vi "Velocidad con Perfiles.vi"() -> ()   [LabVIEW 2014]
uses:
  <vilib>/LabVIEW Interface for Arduino/Type Defs/Pin Mode.ctl
  <vilib>/LabVIEW Interface for Arduino/LabVIEW Interface for Arduino.lvlib
panel:
  out "Boolean 4":bool
  out "Boolean 3":bool
  out "Boolean 2":bool
  out "Boolean":bool
  in  "Enum":enum16{"Detenido", "Baja", "Media", "Alta"}(ring)
  in  "VISA resource name":refnum<visa-resource-name>
  # "Recurso"
  # "Velocidad"
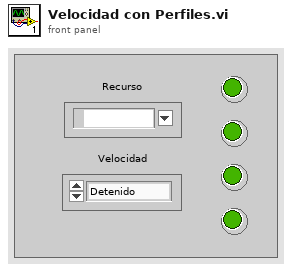
[diagram p1: front panel]
types:
  T1 = typedef "LabVIEW Interface for Arduino.lvlib/Pin Mode.ctl" = enum8{"Input", "Output"}
  T2 = typedef "LabVIEW Interface for Arduino.lvlib/Arduino Resource.ctl" = cluster{"VISA resource":refnum<visa-resource-name>, "Board Type":T3, "Connection Type":enum8{"USB / Serial"}, "Bytes Per Packet (15)":u8}
  T3 = typedef "LabVIEW Interface for Arduino.lvlib/Board Type.ctl" = enum16{"Uno", "Dimuelanove w/Atmega 328", "Mega 2560"}
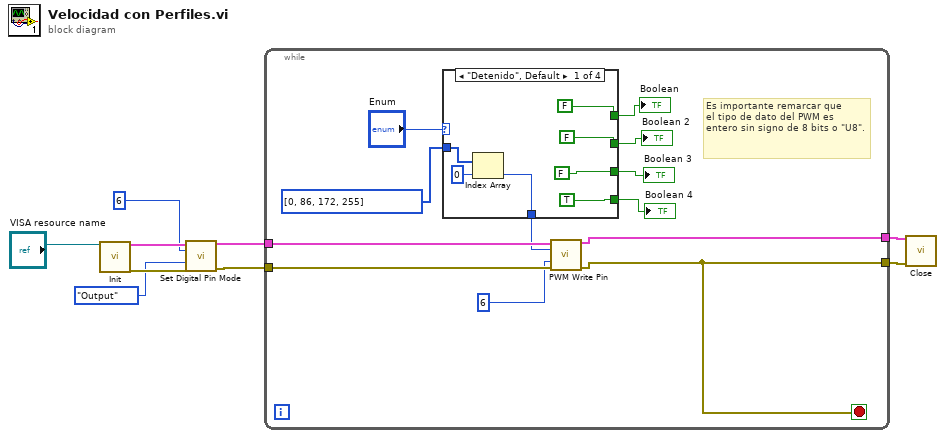
[diagram p0: block diagram]
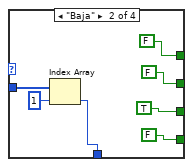
[diagram p2: hidden frame]
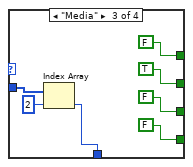
[diagram p3: hidden frame]
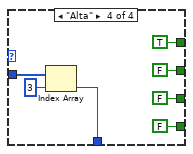
[diagram p4: hidden frame]
diagram:
  n1 = call <vilib>:"Init.vi"("VISA resource"="VISA resource name") -> ("Arduino Resource"=w6:T2, "error out"=w9:errorcluster)  [unwired: 17 in]
  n2 = call <vilib>:"Set Digital Pin Mode.vi"("Arduino Resource"=w6, "Digital I/O Pin"=u8 6, "Pin Mode (Input)"=Pin_Mode."Output", "error in"=w9) -> ("Arduino Resource"=w5:T2, "error out"=w8:errorcluster)  [unwired: 10 in]
  n3 = while {
    tunnel: w8 -> [w21]
    tunnel: [w10] -> w7
    tunnel: w5 -> [w20]
    tunnel: [w19] -> w4
    stop <- w10 stop-if-true
    # "Es importante remarcar que\nel tipo de dato del PWM es entero sin signo de 8 bits o \"U8\"."
    n4 = case shown="\"Detenido\", Default" "Enum" {
      tunnel: [TRUE FALSE FALSE FALSE] -> w16
      tunnel: [FALSE TRUE FALSE FALSE] -> w15
      tunnel: [FALSE FALSE TRUE FALSE] -> w14
      tunnel: [FALSE FALSE FALSE TRUE] -> w13
      tunnel: [w24 w29 w36 w49] -> w12
      tunnel: u8[] [0, 86, 172, 255] -> [w23 w31 w38 w48]
      frame "Detenido", Default {
        n5 = Index Array(array=w23, index=0) -> (element=w24:u8)
      }
      frame "Baja" {
        n6 = Index Array(array=w31, index=1) -> (element=w29:u8)
      }
      frame "Media" {
        n7 = Index Array(array=w38, index=2) -> (element=w36:u8)
      }
      frame "Alta" {
        n8 = Index Array(array=w48, index=3) -> (element=w49:u8)
      }
    }
    "Boolean 4" <- w16
    "Boolean" <- w13
    "Boolean 2" <- w14
    "Boolean 3" <- w15
    n9 = call <vilib>:"PWM Write Pin.vi"("Arduino Resource"=w20, "Duty Cycle (0 - 255)"=w12, "PWM Pin (3)"=u8 6, "error in"=w21) -> ("Arduino Resource"=w19:T2, "error out"=w10:errorcluster)  [unwired: 10 in]
  }
  n10 = call <vilib>:"Close.vi"("Arduino Resource"=w4, "error in"=w7) -> ()  [unwired: 13 in, 1 out]
